vi "ReadDOPin.vi"(8 "error in (no error)":errorcluster, 10 "Pin Number":i32, 11 "connection ID":refnum<k5>) -> (0 "error out":errorcluster, 2 "Port Value":i32, 3 "connection ID out":refnum<k5>)   [LabVIEW 2023, in "Numato.lvlib"]
uses:
  Numato.lvlib
  54457070-54e2-4577-a87b-8c56f91f1dee.vi
panel:
  out "data out":string
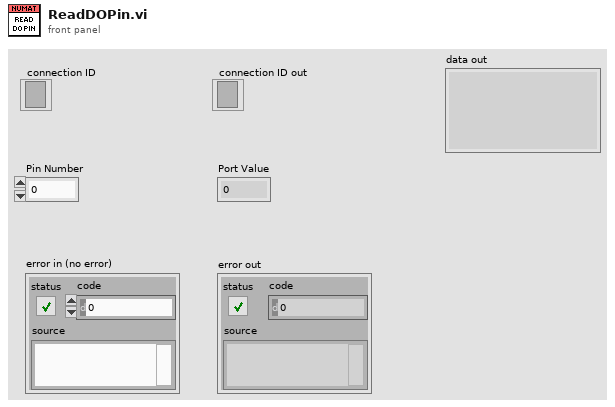
[diagram p1: front panel]
types:
  T1 = enum16{"Standard", "Buffered", "CRLF", "Immediate"}
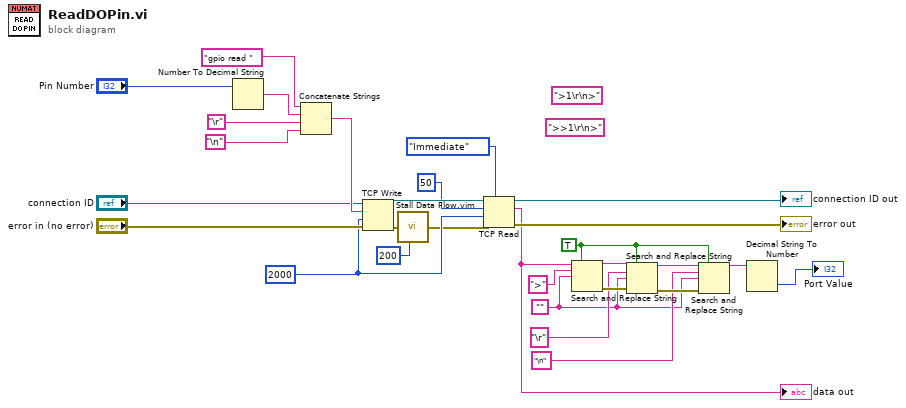
[diagram p0: block diagram]
diagram:
  (unwired) ">>1\r\n>" ("data out")
  w3 = TRUE ("replace all? (F)")
  w4 = ""
  (unwired) ">1\r\n>" ("data out")
  w21 = 2000 ("timeout ms (25000)")
  n1 = Number To Decimal String(number="Pin Number") -> (decimal integer string=w16:string)  [unwired: 1 in]
  n2 = Concatenate Strings("gpio read " ("data in"), w16, "\r", "\n") -> (w27:string)
  n3 = TCP Write(connection ID="connection ID", data in=w27, error in (no error)="error in (no error)", 9:w21) -> (connection ID out=w24:refnum<k5>, error out=w23:errorcluster)  [unwired: 1 out]
  n4 = call "Stall Data Flow.vim"("value in"=w23, "milliseconds to wait"=u32 200) -> ("value out"=w14:errorcluster)  [unwired: 1 out]
  n5 = TCP Read(connection ID=w24, bytes to read=50, error in (no error)=w14, 7:T1."Immediate" ("mode (standard)"), 9:w21) -> (connection ID out=→"connection ID out":refnum<k5>, data out=w12:string, error out=→"error out":errorcluster)
  "data out" <- w12
  n6 = Search and Replace String(replace all?=w3, input string=w12, search string=">" ("data out"), replace string=w4) -> (result string=w10:string, error out=w9:errorcluster)  [unwired: 4 in, 2 out]
  n7 = Search and Replace String(replace all?=w3, input string=w10, search string="\r" ("data out"), replace string=w4, error in=w9) -> (result string=w7:string, error out=w6:errorcluster)  [unwired: 3 in, 2 out]
  n8 = Search and Replace String(replace all?=w3, input string=w7, search string="\n" ("data out"), replace string=w4, error in=w6) -> (result string=w2:string)  [unwired: 3 in, 3 out]
  n9 = Decimal String To Number(string=w2) -> (number=→"Port Value":i32)  [unwired: 2 in, 1 out]
